vi "PAN_GetMods.vi"(9 "Mods dir":path, 10 "configuration file path":path, 11 "Mods In":string[](array[string])=["GUNSC", "GFITS", "LOGIC", "BUFMGR"]) -> (2 "Translations":string[][](array[string]), 3 "Mods Out":string[](array[string]))   [LabVIEW 2016]
uses:
  <vilib>/Utility/config.llb/Read Key (String).vi
  <vilib>/Utility/config.llb/Read Key (Path).vi
  <vilib>/Utility/config.llb/NI_LVConfig.lvlib
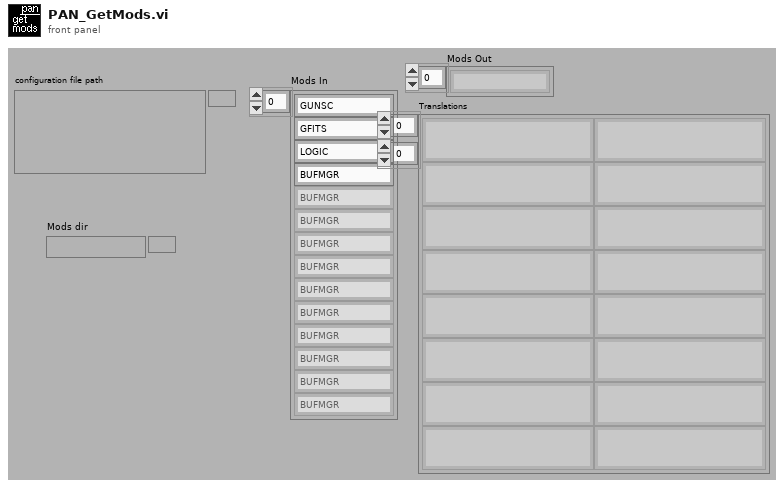
[diagram p1: front panel]
types:
  T1 = typedef "NI_LVConfig.lvlib/Config Data RefNum.ctl" = refnum<k1>
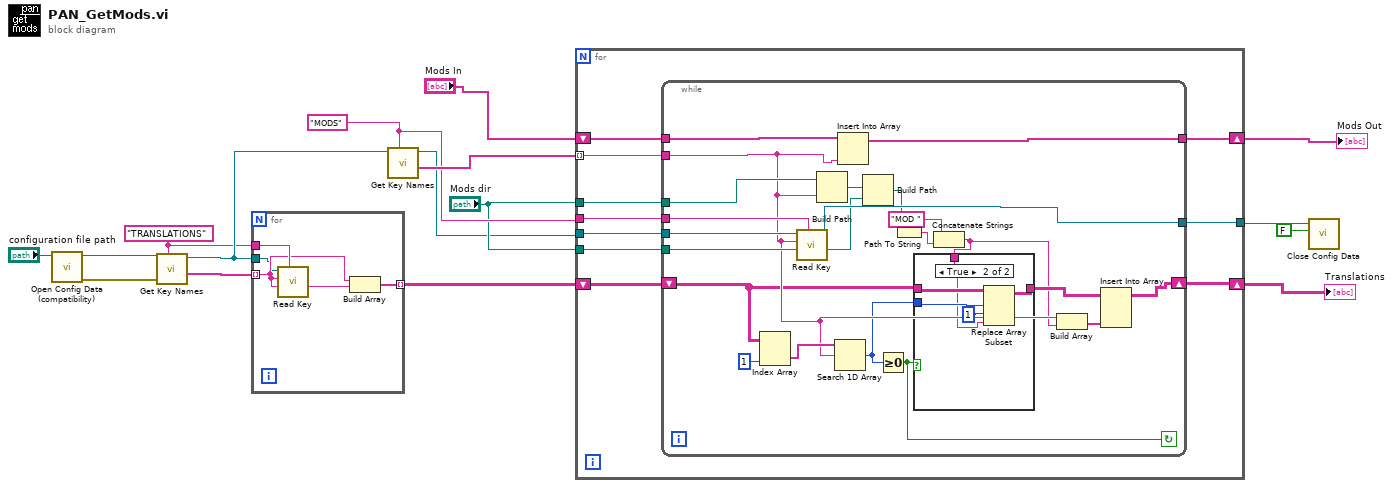
[diagram p0: block diagram]
diagram:
  w3 = "TRANSLATIONS" ("section")
  w13 = "MODS" ("section")
  n1 = call <vilib>:"Open Config Data (compatibility).vi"("configuration file path"="configuration file path") -> ("error out"=w1:errorcluster, "refnum"=w2:T1)  [unwired: 8 in, 1 out]
  n2 = call <vilib>:"Get Key Names.vi"("section"=w3, "error in (no error)"=w1, "refnum"=w2) -> ("key names"=w4:string[], "refnum out"=w8:T1)  [unwired: 7 out]
  n3 = for {
    tunnel: w4 -> [w20] mode=indexing
    tunnel: w8 -> [w17]
    tunnel: w3 -> [w21]
    tunnel: [w18] -> w9 mode=indexing
    n4 = call-poly <vilib>:"Read Key.vi"("section"=w21, "default value"=w20, "key"=w20, "refnum"=w17) -> ("value"=w19:string)  [unwired: 2 in, 5 out]
    n5 = Build Array(w20, w19) -> (w18:string[])
  }
  n6 = call <vilib>:"Get Key Names.vi"("section"=w13, "refnum"=w8) -> ("key names"=w15:string[], "refnum out"=w11:T1)  [unwired: 1 in, 7 out]
  n7 = for {
    tunnel: w15 -> [w24] mode=indexing
    shift-right: [w30] -> w14
    shift-left: "Mods In" -> [w31]
    tunnel: "Mods dir" -> [w25]
    tunnel: w11 -> [w29]
    tunnel: w13 -> [w28]
    tunnel: [w27] -> w10
    tunnel: "Mods dir" -> [w26]
    shift-right: [w23] -> w6
    shift-left: w9 -> [w22]
    n8 = while {
      tunnel: w31 -> [w53]
      tunnel: [w52] -> w30
      tunnel: w29 -> [w51]
      tunnel: w28 -> [w50]
      tunnel: [w49] -> w27
      tunnel: w26 -> [w48]
      tunnel: w25 -> [w47]
      tunnel: w24 -> [w41]
      shift-right: [w34] -> w23
      shift-left: w22 -> [w33]
      stop <- w32 continue-if-true
      n9 = Index Array(array=w33, index (col)=1 ("disabled index (col)")) -> (element=w42:string[])  [unwired: 1 in]
      n10 = call-poly <vilib>:"Read Key.vi"("section"=w50, "default value"=w48, "key"=w41, "refnum"=w51) -> ("value"=w45:path, "refnum out"=w49:T1)  [unwired: 1 in, 5 out]
      n11 = Build Path(base path=w47, name or relative path=w41) -> (appended path=w46:path)
      n12 = Search 1D Array(1D array=w42, element=w41) -> (index of element=w38:i32)  [unwired: 1 out]
      n13 = Insert Into Array(array=w53, new element=w41) -> (w52:string[])  [unwired: 1 in]
      n14 = Build Path(base path=w46, name or relative path=w45) -> (appended path=w44:path)
      n15 = Greater Or Equal To 0?(x=w38) -> (x >= 0?=w32:bool)
      n16 = Path To String(path=w44) -> (string=w37:string)
      n17 = Concatenate Strings("MOD " ("string"), w37) -> (w36:string)
      n18 = case shown="True" w32 {
        tunnel: w33 -> [w54 w59]
        tunnel: [w54 w56] -> w39
        tunnel: w38 -> [_ w58]
        tunnel: w36 -> [_ w55]
        frame False {
        }
        frame True {
          n19 = Replace Array Subset(array=w59, new element=w55, index (row)=w58, index (col)=1 ("disabled index (col)")) -> (w56:string[][])
        }
      }
      n20 = Build Array(w41, w36) -> (w40:string[])
      n21 = Insert Into Array(array=w39, new element=w40) -> (w34:string[][])  [unwired: 2 in]
    }
  }
  "Mods Out" <- w14
  "Translations" <- w6
  n22 = call <vilib>:"Close Config Data.vi"("write file if changed (T)"=FALSE ("write configuration file? (T)"), "refnum"=w10) -> ()  [unwired: 1 in, 9 out]
